vi "apply data indices.vi"(8 "error in":errorcluster, 9 "index cluster":variant, 10 "channel classification":T1, 11 "System Diagnostics runtime in":refnum<class "System Diagnostics runtime.lvclass">) -> (0 "error out":errorcluster, 3 "System Diagnostics runtime out":refnum<class "System Diagnostics runtime.lvclass">)   [LabVIEW 2013, in "System Diagnostics runtime.lvclass"]
uses:
  System Diagnostics runtime.lvclass
  <vilib>/NI/Tag Bus Module Framework/channel/channel classification.ctl
  configuration/input data indices.ctl
  System Diagnostics runtime.lvclass/System Diagnostics runtime.ctl
  configuration/System Diagnostics configuration.lvclass
  <vilib>/NI/Tag Bus Module Framework/channel/TBM channel.lvclass
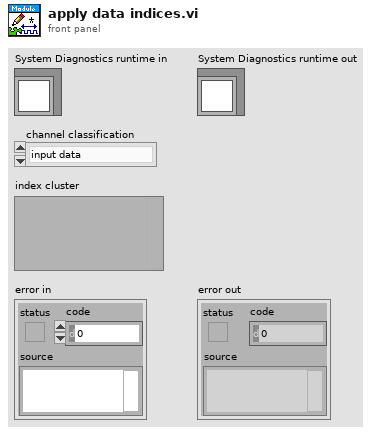
[diagram p1: front panel]
types:
  T1 = typedef "TBM channel.lvclass/channel classification.ctl" = enum16{"input data", "output data", "processing parameter", "processing result"}
  T2 = typedef "System Diagnostics configuration.lvclass/input data indices.ctl" = cluster{"Double.CPU load average":i32, "Double.timed structures load":i32, "Double.free memory":i32, "Double.contiguous memory":i32}
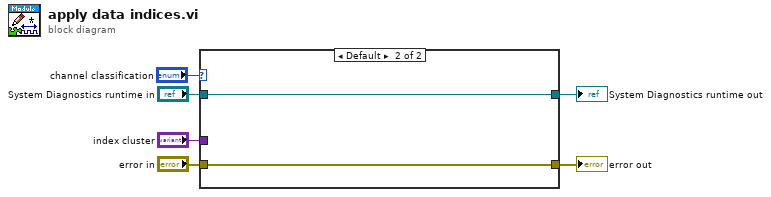
[diagram p0: block diagram]
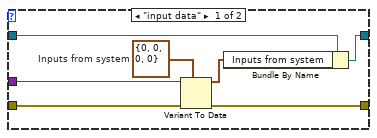
[diagram p2: hidden frame]
diagram:
  n1 = case shown="Default" "channel classification" {
    tunnel: "index cluster" -> [w11 _]
    tunnel: [w10 w15] -> w4
    tunnel: "System Diagnostics runtime in" -> [w9 w15]
    tunnel: "error in" -> [w8 w14]
    tunnel: [w7 w14] -> w1
    frame "input data" {
      w13 = T2 {"Double.CPU load average"=0, "Double.timed structures load"=0, "Double.free memory"=0, "Double.contiguous memory"=0}  # Inputs from system
      n2 = Variant To Data(error in=w8, type=w13, Variant=w11) -> (data=w12:T2, error out=w7:errorcluster)
      n3 = Bundle By Name(cluster=w9, "Inputs from system"=w12) -> (w10:refnum<class "System Diagnostics runtime.lvclass">)
    }
    frame Default {
    }
  }
  "error out" <- w1
  "System Diagnostics runtime out" <- w4
